vi "Gatilho de aquisição em linha.vi"() -> ()   [LabVIEW 2020]
uses:
  <vilib>/vision/Measure.llb/Edge New.ctl
  <vilib>/vision/Image Controls.llb/IMAQ Image.ctl
panel:
  in  "Image In":T1
  out "Salvando peças":bool
  out "Peça detectada":bool
  out "Image":T1(plugin-control)
  out "Edge Information (Edge Detector 1)":T2[](array[typedef]) {"Distance (Real-World)" format="%.2f"; "Location (Real-World)"."Y" format="%.2g"; "Location (Real-World)"."X" format="%.2f"; "Noise" format="%.2f"; "Location (Pixel)"."Y" format="%.2g"; "Location (Pixel)"."X" format="%.2f"; "Strength" format="%.2f"; "Distance (Pixel)" format="%.2f"}
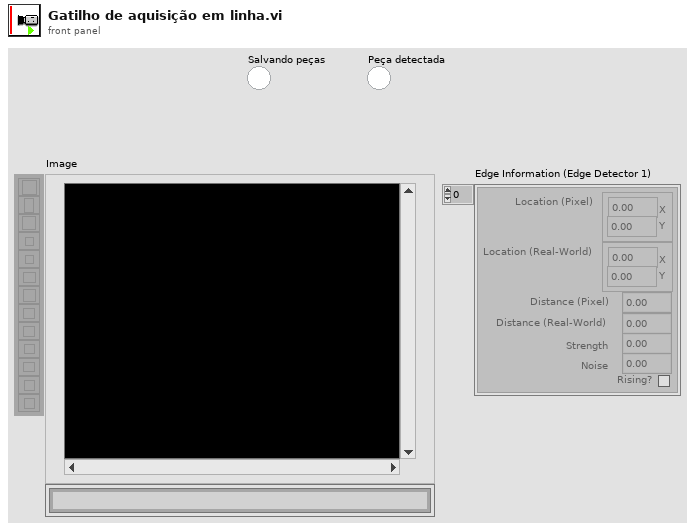
[diagram p1: front panel]
types:
  T1 = typedef "IMAQ Image.ctl" = refnum<image>
  T2 = typedef "Edge New.ctl" = cluster{"Location (Pixel)":cluster{"X":sgl, "Y":sgl}, "Location (Real-World)":cluster{"X":sgl, "Y":sgl}, "Distance (Pixel)":dbl, "Distance (Real-World)":dbl, "Strength":dbl, "Noise":dbl, "Rising?":bool}
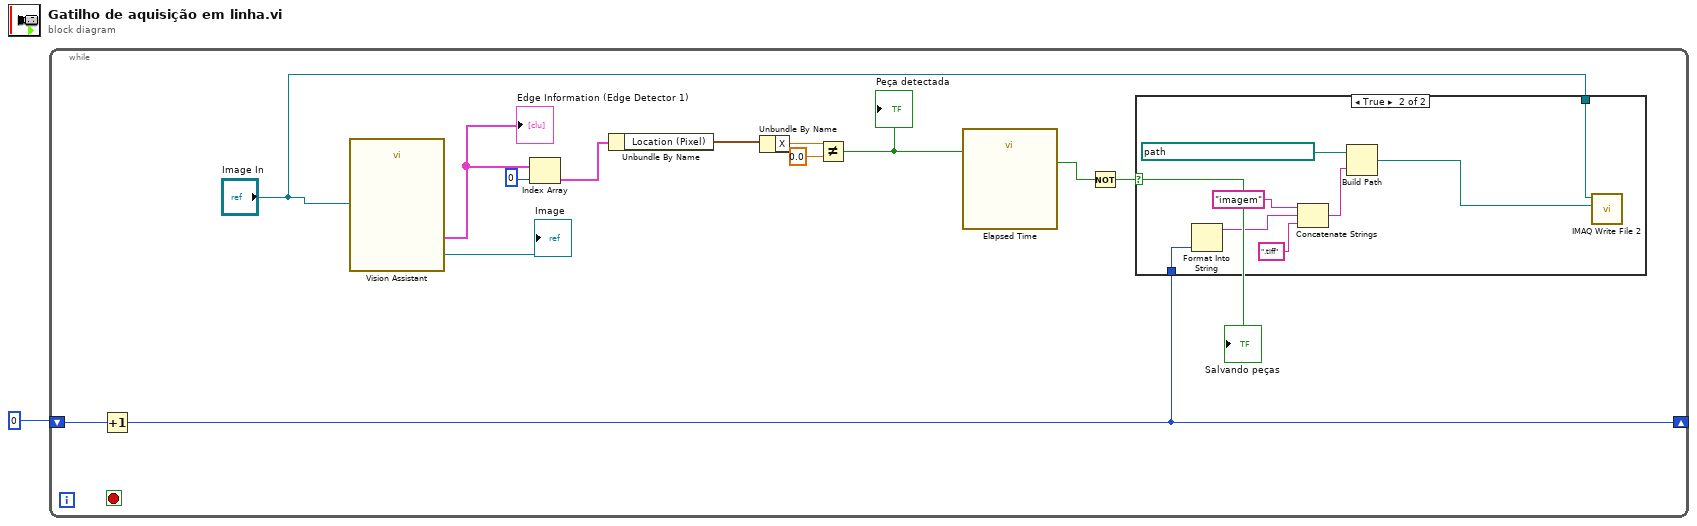
[diagram p0: block diagram]
diagram:
  n1 = while {
    shift-right: [w3] -> _
    shift-left: 0 -> [w4]
    stop <- _ stop-if-true
    n2 = Increment(x=w4) -> (x+1=w3:i32)
    n3 = call "Vision Assistant"("Image In"="Image In") -> ("Image Out"=→"Image":T1, "Edge Information (Edge Detector 1)"=w13:T2[])  [unwired: 24 in, 1 out]
    "Edge Information (Edge Detector 1)" <- w13
    n4 = Index Array(array=w13, index=0) -> (element=w11:T2)
    n5 = Unbundle By Name(w11) -> ("Location (Pixel)"=w10:cluster{"X":sgl, "Y":sgl})
    n6 = Unbundle By Name(w10) -> ("X"=w9:sgl)
    n7 = Not Equal?(x=w9, y=sgl 0.0) -> (x != y?=w7:bool)
    "Peça detectada" <- w7
    n8 = call "Elapsed Time"("Reset"=w7) -> ("Time has Elapsed"=w6:bool)  [unwired: 11 in, 7 out]
    n9 = Not(x=w6) -> (.not. x?=w5:bool)
    "Salvando peças" <- w5
    n10 = case shown="True" w5 {
      tunnel: "Image In" -> [_ w22]
      tunnel: w3 -> [_ w19]
      frame False {
      }
      frame True {
        n11 = Format Into String(w19) -> (resulting string=w18:string)  [unwired: 3 in, 1 out]
        n12 = Concatenate Strings("imagem" ("string"), w18, ".tiff" ("string")) -> (w16:string)
        n13 = Build Path(base path=path "C:/Users/Beneli/Desktop/peça", name or relative path=w16) -> (appended path=w15:path)
        n14 = call-poly "IMAQ Write File 2"("File Path"=w15, "Image"=w22) -> ()  [unwired: 8 in, 2 out]
      }
    }
  }
